vi "Write Serial Number.vi"(8 "error in (no error)":errorcluster, 10 "Serial Number":u16, 11 "CCDCamera in":refnum<class "CCDCamera.lvclass">) -> (0 "error out":errorcluster, 3 "CCDCamera out":refnum<class "CCDCamera.lvclass">)   [LabVIEW 2018, in "CCDCamera.lvclass"]
uses:
  CCDCamera.lvclass
  CCDCamera.lvclass/CCDCamera.ctl
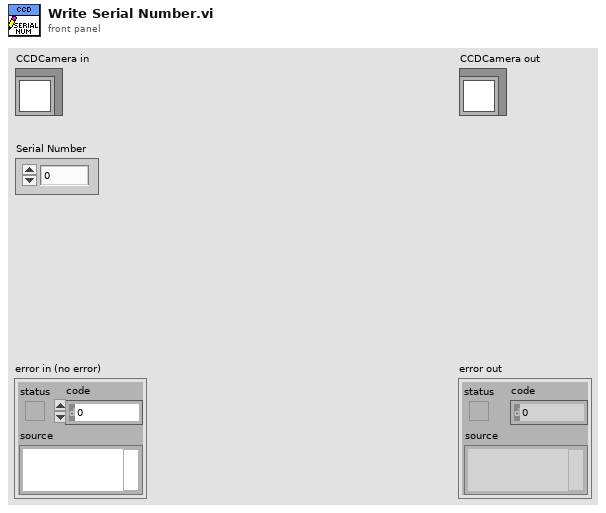
[diagram p1: front panel]
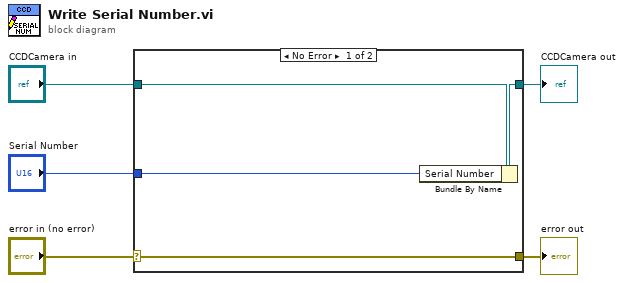
[diagram p0: block diagram]
diagram:
  n1 = case shown="No Error" "error in (no error)" {
    selector: "error in (no error)" -> [w9 w10]
    tunnel: [w9 w10] -> w4
    tunnel: [w7 w11] -> w2
    tunnel: "CCDCamera in" -> [w8 w11]
    tunnel: "Serial Number" -> [w6 _]
    frame No Error {
      n2 = Bundle By Name(cluster=w8, "Serial Number"=w6) -> (w7:refnum<class "CCDCamera.lvclass">)
    }
    frame Error {
    }
  }
  "error out" <- w4
  "CCDCamera out" <- w2
